vi "Write Static System Messenger.vi"(8 "error in (no error)":errorcluster, 10 "Messenger.lvclass":refnum<class "Messenger.lvclass">, 11 "Root Actor in":refnum<class "Root Actor.lvclass">) -> (0 "error out":errorcluster, 3 "Root Actor out":refnum<class "Root Actor.lvclass">)   [LabVIEW 2024, in "Root Actor.lvclass"]
uses:
  Root Actor.lvclass
  Messenger/Messenger/Messenger.lvclass
  Root Actor.lvclass/Root Actor.ctl
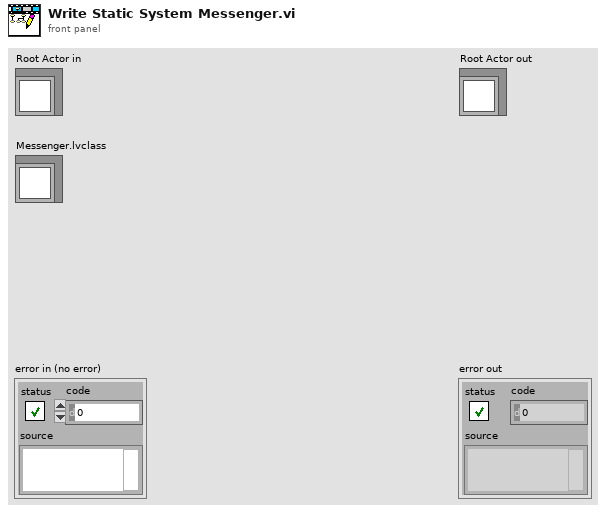
[diagram p1: front panel]
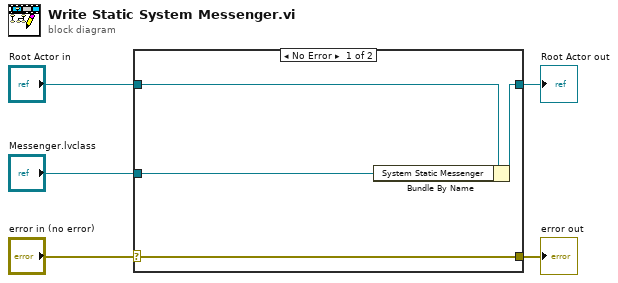
[diagram p0: block diagram]
diagram:
  n1 = case shown="No Error" "error in (no error)" {
    selector: "error in (no error)" -> [w9 w10]
    tunnel: [w9 w10] -> w4
    tunnel: [w7 w11] -> w2
    tunnel: "Root Actor in" -> [w8 w11]
    tunnel: "Messenger.lvclass" -> [w6 _]
    frame No Error {
      n2 = Bundle By Name(cluster=w8, "System Static Messenger"=w6) -> (w7:refnum<class "Root Actor.lvclass">)
    }
    frame Error {
    }
  }
  "error out" <- w4
  "Root Actor out" <- w2
